vi "Main_Task.vi"(8 "error in (no error)":errorcluster, 10 "DS Occurence":refnum<k4>, 11 "Autonomous VI in":refnum<vi>) -> ()   [LabVIEW 2011]
uses:
  script/Auto_Conf.vi
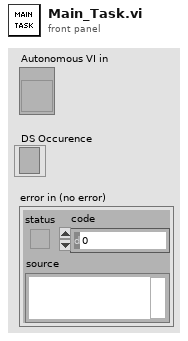
[diagram p1: front panel]
types:
  T1 = enum16{"push_data", "write_joe_johnson", "write_roller", "write_drivetrain", "write_gun_fast", "write_gun_slow"}
  T2 = typedef "WPI_DriverStationDerivedRobotMode.ctl" = enum16{"Init", "Execute", "Stop"}
  T3 = typedef "WPI_DriverStationRobotMode.ctl" = enum16{"Autonomous Disabled", "Autonomous Enabled", "Teleop Disabled", "Teleop Enabled", "Timeout", "Finish"}
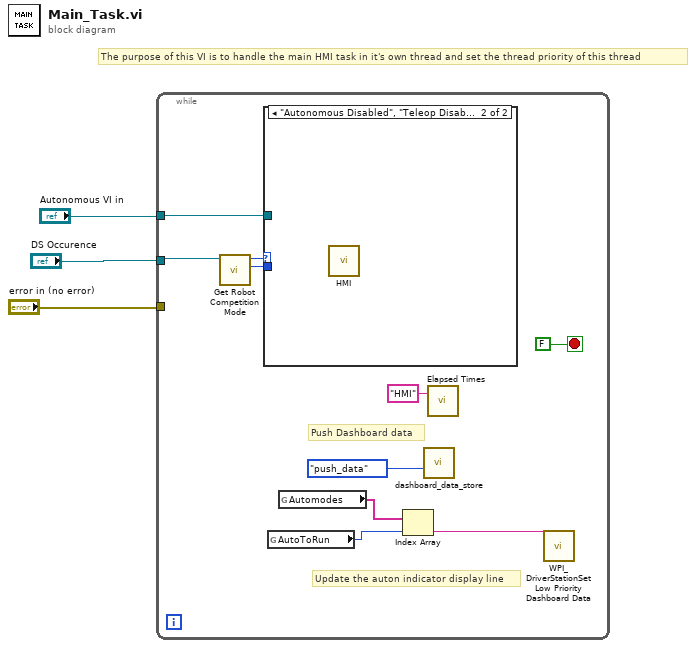
[diagram p0: block diagram]
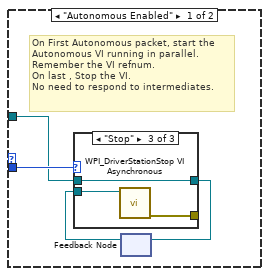
[diagram p2: hidden frame]
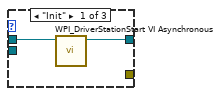
[diagram p3: hidden frame]
diagram:
  # "The purpose of this VI is to handle the main HMI task in it's own thread and set the thread priority of this thread"
  n1 = while {
    tunnel: "DS Occurence" -> [w11]
    tunnel: "error in (no error)" -> [_]
    tunnel: "Autonomous VI in" -> [w10]
    stop <- FALSE stop-if-true
    # "Update the auton indicator display line"
    # "Push Dashboard data"
    n2 = call "Get Robot Competition Mode.vi"("DS Occurrence"=w11) -> ("Call Context"=w13:T2, "Robot Mode"=w12:T3)  [unwired: 1 in, 8 out]
    n3 = case shown="\"Autonomous Disabled\", \"Teleop Disabled\", \"Teleop Enabled\", Default" w12 {
      tunnel: w13 -> [w17 _]
      tunnel: w10 -> [w16 _]
      frame "Autonomous Enabled" {
        # "On First Autonomous packet, start the\nAutonomous VI running in parallel.\nRemember the VI refnum.\nOn last , Stop the VI.\nNo need to respond to intermediates."
        n4 = feedback #1() -> (w14:refnum<vi>)  [unwired: 1 out]
        n5 = case shown="\"Stop\"" w17 {
          tunnel: w16 -> [w19 _ w22]
          tunnel: [w18 w20 w22] -> w15
          tunnel: w14 -> [_ w20 w23]
          tunnel: [_ _ w21] -> _
          frame "Init" {
            n6 = call <vilib>:"WPI_DriverStationStart VI Asynchronous.vi"("VI"=w19) -> ("VI out"=w18:refnum<vi>)  [unwired: 10 out]
          }
          frame "Execute", Default {
            # "Nothing to do"
          }
          frame "Stop" {
            n7 = call <vilib>:"WPI_DriverStationStop VI Asynchronous.vi"("VI Refnum"=w23) -> ("error out"=w21:errorcluster)  [unwired: 10 out]
          }
        }
        n8 = feedback-in #1(w15) -> ()
      }
      frame "Autonomous Disabled", "Teleop Disabled", "Teleop Enabled", Default {
        n9 = call "HMI.vi"() -> ()  [unwired: 3 in, 9 out]
      }
    }
    n10 = global read "Auto_Conf.vi" "AutoToRun"() -> (w6:u8)
    n11 = global read "Auto_Conf.vi" "Automodes"() -> (w7:string[])
    n12 = Index Array(array=w7, index=w6) -> (element=w5:string)
    n13 = call "dashboard_data_store.vi"("mode"=T1."push_data") -> ()  [unwired: 11 in]
    n14 = call "Elapsed Times.vi"("Call Name"="HMI") -> ()  [unwired: 2 in, 1 out]
    n15 = call <vilib>:"WPI_DriverStationSet Low Priority Dashboard Data.vi"("User Data"=w5) -> ()  [unwired: 10 in, 1 out]
  }
